vi "L01P1-1.vi"() -> ()   [LabVIEW 2011]
doc: "Use this template to generate a signal and display the generated data in a graph. You can use this template with the exercises in the Getting Started with LabVIEW manual.\nNote: LabVIEW enables automatic error handling by default for VIs you create from this template."
uses:
  Instance           1 35Saved   TutorialGenerateDisplay.vit .vi
panel:
  in  "Numeric":dbl
  in  "Knob":dbl(knob) scale=0.0..10.0
  out "Waveform Graph":dynamicdata(graph)
  in  "stop":bool
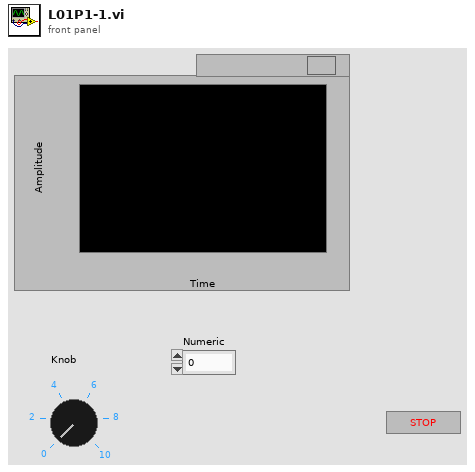
[diagram p1: front panel]
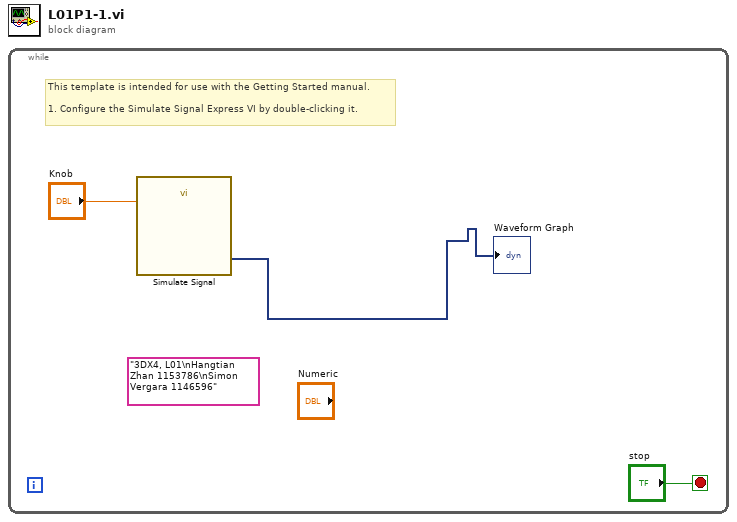
[diagram p0: block diagram]
diagram:
  n1 = while {
    stop <- "stop" stop-if-true
    (unwired) "3DX4, L01\nHangtian Zhan 1153786\nSimon Vergara 1146596"
    # "This template is intended for use with the Getting Started manual.\n\n1. Configure the Simulate Signal Express VI by double-clicking it."
    n2 = call "Simulate Signal"("Amplitude"="Knob") -> ("Sawtooth"=→"Waveform Graph":dynamicdata)  [unwired: 13 in, 1 out]
  }
